vi "DriveGetSpeed.vi"() -> (0 "Right speed (ft/s)":dbl, 1 "Left speed (ft/s)":dbl)   [LabVIEW 2020]
doc: "Get speed variable for drive \n\nOutput\n-- Left Speed -- Double -- Speed of left drive train, based on encoder values --\n-- Right Speed -- Double -- Speed of right train, based on encoder values--"
uses:
  DriveGlobal.vi
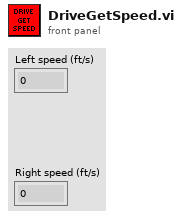
[diagram p1: front panel]
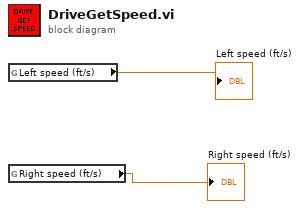
[diagram p0: block diagram]
diagram:
  n1 = global read "DriveGlobal.vi" "Left speed (ft/s)"() -> (→"Left speed (ft/s)":dbl)
  n2 = global read "DriveGlobal.vi" "Right speed (ft/s)"() -> (→"Right speed (ft/s)":dbl)
